vi "group Bulk Read Get Data.vi"(7 "data_length":u16, 8 "error in (no error)":errorcluster, 9 "address":u16, 10 "id":u8, 11 "group_num":i32) -> (0 "error out":errorcluster, 3 "function return":u32)   [LabVIEW 2018, in "labview.lvlib"]
doc: "WINDECLSPEC uint32_t groupBulkReadGetData (int group_num, uint8_t id, uint16_t address, uint16_t data_length);"
uses:
  labview.lvlib
  dxl_x86_c.dll
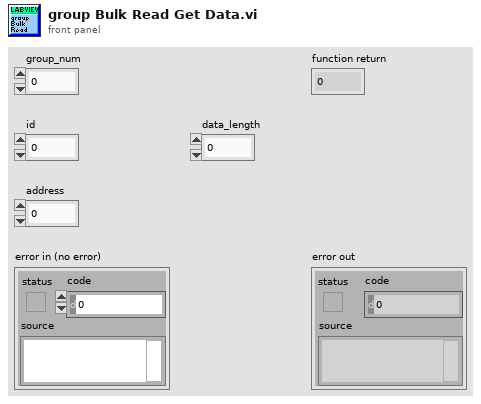
[diagram p1: front panel]
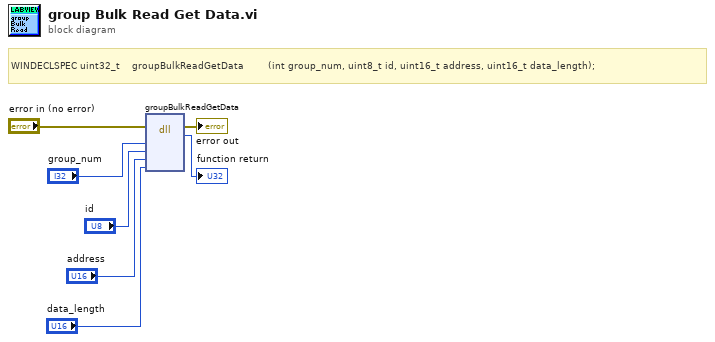
[diagram p0: block diagram]
diagram:
  # "WINDECLSPEC uint32_t    groupBulkReadGetData        (int group_num, uint8_t id, uint16_t address, uint16_t data_length);"
  n1 = dll-call lib="C:/Users/joaos/OneDrive/Documents/[PhD]/Project Omnidirectional Vehicle/Vanes/LabView_code/joaoandthethreestands/DynamixelSDK-3.7.31/labview/new_compilation/dxl_x86_c.*" fn="groupBulkReadGetData"(error in="error in (no error)", "group_num"="group_num", "id"="id", "address"="address", "data_length"="data_length") -> (error out=→"error out":errorcluster, →"function return":u32)  [unwired: 6 in, 1 out]
